vi "DeleteTerminal.vi"(8 "error in (no error)":errorcluster, 11 "Refnum TerminalToDelete":refnum<vi>) -> (0 "error out":errorcluster)   [LabVIEW 2011]
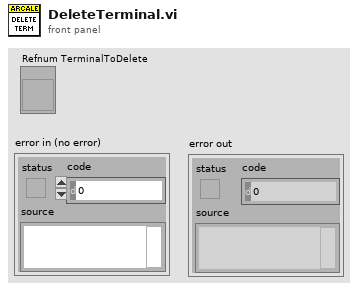
[diagram p1: front panel]
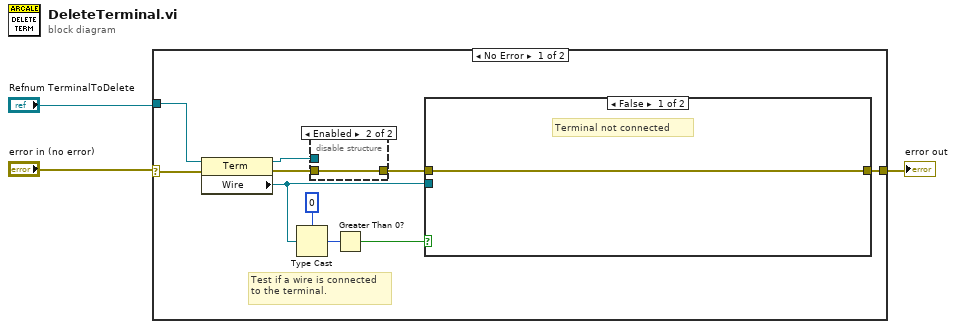
[diagram p0: block diagram]
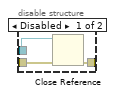
[diagram p2: hidden frame]
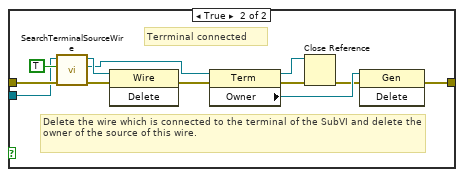
[diagram p3: hidden frame]
diagram:
  n1 = case shown="No Error" "error in (no error)" {
    selector: "error in (no error)" -> [w13 w31]
    tunnel: [w12 w31] -> w2
    tunnel: "Refnum TerminalToDelete" -> [w11 _]
    frame No Error {
      # "Test if a wire is connected to the terminal."
      n2 = property class="Term"(reference=w11, error in=w13) -> (reference out=w4:refnum<vi>, error out=w6:errorcluster, "Wire"=w8:refnum<vi>)
      n3 = Type Cast(type=u32 0 ("index"), x=w8) -> (*(type *) &x=w9:u32)
      n4 = disable-structure shown="Enabled" {
        disable-tunnel: w6 -> [w16 w17]
        disable-tunnel: [w15 w17] -> w5
        disable-tunnel: w4 -> [w14 _]
        frame Disabled {
          n5 = Close Reference(reference=w14, error in (no error)=w16) -> (error out=w15:errorcluster)
        }
        frame Enabled {
        }
      }
      n6 = Greater Than 0?(x=w9) -> (x > 0?=w7:bool)
      n7 = case shown="False" w7 {
        tunnel: w5 -> [w18 w30]
        tunnel: [w18 w23] -> w12
        tunnel: w8 -> [_ w22]
        frame False {
          # "Terminal not connected"
        }
        frame True {
          # "Delete the wire which is connected to the terminal of the SubVI and delete the owner of the source of this wire."
          # "Terrminal connected"
          n8 = call "SearchTerminalSourceWire.vi"("error in (no error)"=w30, "Source?"=TRUE, "Refnum Wire In"=w22) -> ("error out"=w27:errorcluster, "Terminal Refnum"=w25:refnum<vi>, "Refnum Wire Out"=w26:refnum<vi>)  [unwired: 6 in]
          n9 = invoke class="Wire" method="Delete"(reference=w26, error in=w27) -> (error out=w24:errorcluster)  [unwired: 1 in, 2 out]
          n10 = property class="Term"(reference=w25, error in=w24) -> (reference out=w19:refnum<vi>, error out=w21:errorcluster, "Owner"=w29:refnum<vi>)
          n11 = Close Reference(reference=w19, error in (no error)=w21) -> (error out=w20:errorcluster)
          n12 = invoke class="Gen" method="Delete"(reference=w29, error in=w20) -> (error out=w23:errorcluster)  [unwired: 1 in, 2 out]
        }
      }
    }
    frame Error {
    }
  }
  "error out" <- w2
